vi "LoadConfig.vi"(6 "error in (no error)":errorcluster, 8 "Start and End":T1, 9 "Array":path[](array[path])) -> (0 "error out":errorcluster, 3 "data":string[][][](array[string]))   [LabVIEW 2014]
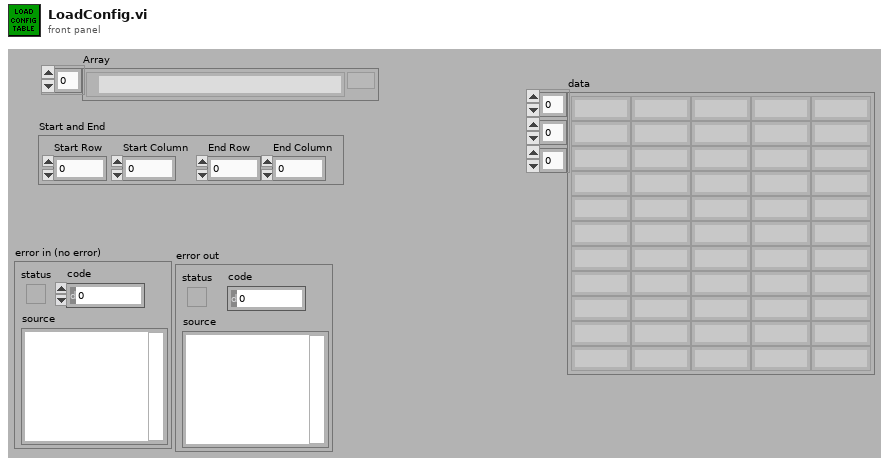
[diagram p1: front panel]
types:
  T1 = cluster{"Start Row":i32, "Start Column":i32, "End Row":i32, "End Column":i32}
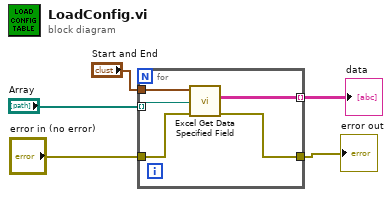
[diagram p0: block diagram]
diagram:
  n1 = for {
    tunnel: "Start and End" -> [w10]
    tunnel: "Array" -> [w9] mode=indexing
    tunnel: [w8] -> w3 mode=indexing
    tunnel: "error in (no error)" -> [w7]
    tunnel: [w6] -> w1
    n2 = call "Excel Get Data Specified Field.vi"("error in (no error)"=w7, "path"=w9, "Start and End"=w10) -> ("error out"=w6:errorcluster, "data"=w8:string[][])  [unwired: 2 in, 1 out]
  }
  "data" <- w3
  "error out" <- w1
